vi "Configure Temperature (Thermistor).vi"(0 "VISA resource name":refnum<visa-resource-name>, 5 "Wire Mode (1: 4-Wire)":i16(ring)=1 items=["2-Wire", "4-Wire"], 7 "Unit (0: Celsius)":u16(ring) items=["C", "F", "K"], 9 "Probe Type (5000)":i16(ring)=5000 items=["2.2k"=2252, "5k"=5000, "10k"=10000], 11 "error in (no error)":errorcluster) -> (4 "VISA resource name out":refnum<visa-resource-name>, 15 "error out":errorcluster)   [LabVIEW 2022 SP3, in "Agilent 34401.lvlib"]
doc: "Configures the settings for a 2-wire or 4-wire thermistor.\n\n<B>Note:</B>\n\nThis VI only applies to the 34410/34411 models."
uses:
  <instrlib>/Agilent 34401/Agilent 34401.lvlib
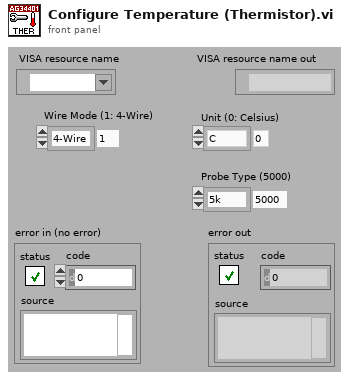
[diagram p1: front panel]
types:
  T1 = typedef "Agilent 34401.lvlib/Extended User Data.ctl" = cluster{"Trigger Source":u16, "Math Storage":u16, "Agilent Model":i32}
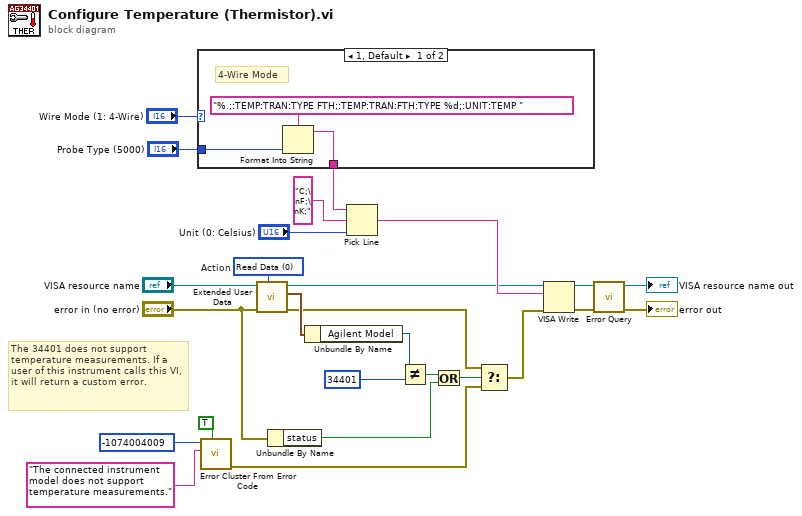
[diagram p0: block diagram]
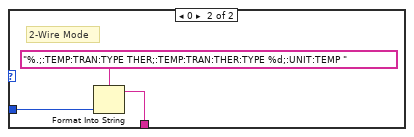
[diagram p2: hidden frame]
diagram:
  w7 = u16 0 items=["Read Data", "Write Data", "Dispose of Data"]  # Action
  # "The 34401 does not support temperature measurements. If a user of this instrument calls this VI, it will return a custom error."
  n1 = case shown="1, Default" "Wire Mode (1: 4-Wire)" {
    tunnel: "Probe Type (5000)" -> [w29 w31]
    tunnel: [w28 w30] -> w19
    frame 1, Default {
      # "4-Wire Mode"
      n2 = Format Into String(format string="%.;:TEMP:TRAN:TYPE FTH;:TEMP:TRAN:FTH:TYPE %d;:UNIT:TEMP ", w29) -> (resulting string=w28:string)  [unwired: 2 in, 1 out]
    }
    frame 0 {
      # "2-Wire Mode"
      n3 = Format Into String(format string="%.;:TEMP:TRAN:TYPE THER;:TEMP:TRAN:THER:TYPE %d;:UNIT:TEMP ", w31) -> (resulting string=w30:string)  [unwired: 2 in, 1 out]
    }
  }
  n4 = call <vilib>:"Error Cluster From Error Code.vi"("show call chain? (False)"=TRUE, "error message (\"\")"="The connected instrument model does not support temperature measurements." ("Source (VI Name)"), "error code (0)"=-1074004009 ("Code")) -> ("error out"=w13:errorcluster)  [unwired: 6 in]
  n5 = call <instrlib>:"Extended User Data.vi"("Action (0: Read Data)"=w7, "Error In (no error)"="error in (no error)", "VISA resource name in"="VISA resource name") -> ("Error Out"=w2:errorcluster, "User Data Out"=w6:T1, "VISA resource name out"=w3:refnum<visa-resource-name>)  [unwired: 6 in]
  n6 = Unbundle By Name("error in (no error)") -> ("status"=w9:bool)
  n7 = Unbundle By Name(w6) -> ("Agilent Model"=w1:i32)
  n8 = Pick Line(string ("")=w19, multi-line string="C;\nF;\nK;", line index="Unit (0: Celsius)") -> (output string=w18:string)
  n9 = Not Equal?(x=w1, y=u32 34401 ("x")) -> (x != y?=w11:bool)
  n10 = Or(x=w11, y=w9) -> (x .or. y?=w10:bool)
  n11 = Select(t=w2, s=w10, f=w13) -> (s? t:f=w12:errorcluster)
  n12 = VISA Write(VISA resource name=w3, write buffer=w18, error in (no error)=w12) -> (VISA resource name out=w24:refnum<visa-resource-name>, error out=w23:errorcluster)  [unwired: 1 out]
  n13 = call <instrlib>:"Error Query.vi"("error in (no error)"=w23, "VISA resource name"=w24) -> ("error out"=→"error out":errorcluster, "VISA resource name out"=→"VISA resource name out":refnum<visa-resource-name>)  [unwired: 6 in, 2 out]
